vi "Api_GetWaveform.vi"(8 "error in (no error)":errorcluster caption="错误输入（无错误）", 11 "Tags[]":string[](array[string])) -> (0 "error out":errorcluster caption="错误输出", 1 "Display?":bool, 2 "Wave[]":waveform(dbl)[](array[waveform]))   [LabVIEW 2016]
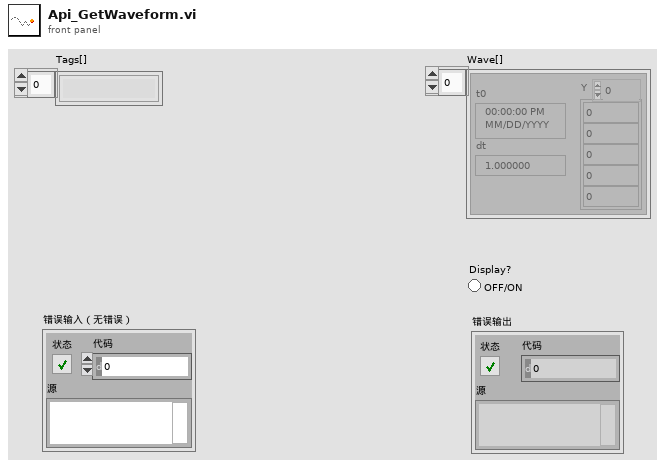
[diagram p1: front panel]
types:
  T1 = cluster{"Queue Name":string, "DAQ Channels":string[], "Queue Type":string}[]
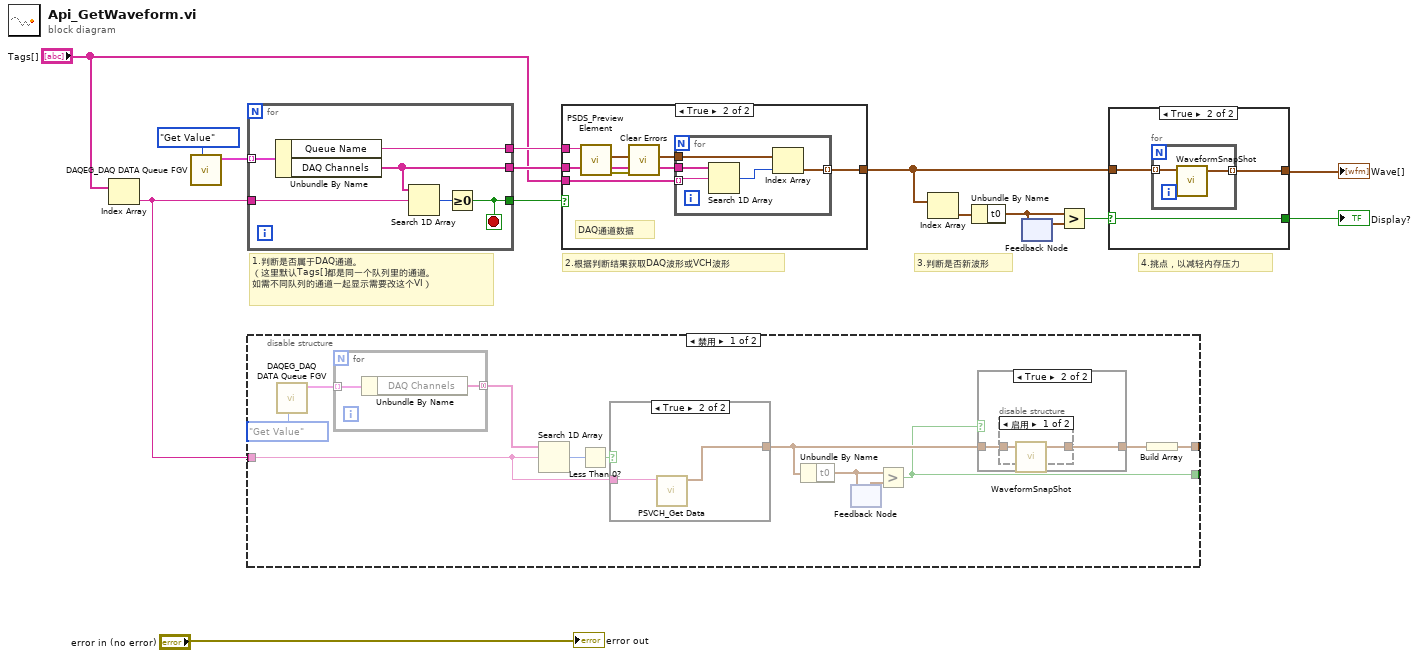
[diagram p0: block diagram]
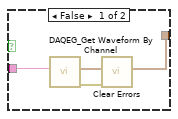
[diagram p2: hidden frame]
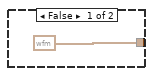
[diagram p3: hidden frame]
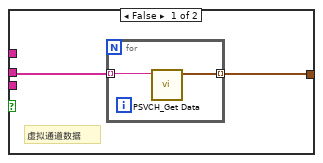
[diagram p7: hidden frame]
diagram:
  # "4.挑点，以减轻内存压力"
  # "3.判断是否新波形"
  # "2.根据判断结果获取DAQ波形或VCH波形"
  # "1.判断是否属于DAQ通道。\n（这里默认Tags[]都是同一个队列里的通道。\n如需不同队列的通道一起显示需要改这个VI）"
  n1 = Index Array(array="Tags[]") -> (element=w12:string)  [unwired: 1 in]
  n2 = call "DAQEG_DAQ DATA Queue FGV.vi"("Command"=enum16{"Initialize", "Get Value", "Set Value"}."Get Value") -> ("DAQ DATA Out"=w13:T1)  [unwired: 9 in, 1 out]
  n3 = for {
    tunnel: w13 -> [w21] mode=indexing
    tunnel: [w20] -> w9
    tunnel: w12 -> [w19]
    tunnel: [w17] -> w11
    tunnel: [w16] -> w10
    stop <- w16 stop-if-true
    n4 = Unbundle By Name(w21) -> ("Queue Name"=w17:string, "DAQ Channels"=w20:string[])
    n5 = Search 1D Array(1D array=w20, element=w19) -> (index of element=w18:i32)  [unwired: 1 in]
    n6 = Greater Or Equal To 0?(x=w18) -> (x >= 0?=w16:bool)
  }
  n7 = disable-structure shown="禁用" {
    disable-tunnel: [w26 _] -> _
    disable-tunnel: [w23 _] -> _
    disable-tunnel: w12 -> [w22 _]
    frame Disabled {
      n8 = call "DAQEG_DAQ DATA Queue FGV.vi"("Command"=enum16{"Initialize", "Get Value", "Set Value"}."Get Value") -> ("DAQ DATA Out"=w27:T1)  [unwired: 9 in, 1 out]
      n9 = for {
        tunnel: w27 -> [w35] mode=indexing
        tunnel: [w34] -> w25 mode=concatenating
        n10 = Unbundle By Name(w35) -> ("DAQ Channels"=w34:string[])
      }
      n11 = Search 1D Array(1D array=w25, element=w22) -> (index of element=w30:i32)  [unwired: 1 in]
      n12 = Less Than 0?(x=w30) -> (x < 0?=w29:bool)
      n13 = case shown="True" w29 {
        tunnel: w22 -> [w38 w40]
        tunnel: [w37 w39] -> w31
        frame False {
          n14 = call "DAQEG_Get Waveform By Channel.vi"("DAQ Channel"=w38) -> ("error out"=w36:errorcluster, "waveform"=w37:waveform(dbl))  [unwired: 9 in]
          n15 = call <vilib>:"Clear Errors.vi"("error in (no error)"=w36) -> ()  [unwired: 5 in, 2 out]
        }
        frame True {
          n16 = call "PSVCH_Get Data.vi"("ChlName"=w40) -> ("Data"=w39:waveform(dbl))  [unwired: 8 in, 2 out]
        }
      }
      n17 = Unbundle By Name(w31) -> ("t0"=w32:timestamp)
      n18 = feedback #1() -> (w33:timestamp)  [unwired: 1 in]
      n19 = feedback-in #1(w32) -> ()
      n20 = Greater?(x=w32, y=w33) -> (0:w26:bool)
      n21 = case shown="True" w26 {
        tunnel: w31 -> [_ w43]
        tunnel: [waveform(dbl) {"t0"=timestamp(0 s since 1904-01-01), "dt"=1.0, "Y"=[]} ("signal out") w42] -> w24
        frame False {
        }
        frame True {
          n22 = disable-structure shown="启用" {
            disable-tunnel: w43 -> [w45 w46]
            disable-tunnel: [w44 w46] -> w42
            frame Enabled {
              n23 = call "WaveformSnapShot.vi"("RawWave"=w45) -> ("SnapWave"=w44:waveform(dbl))  [unwired: 7 in, 1 out]
            }
            frame Disabled {
            }
          }
        }
      }
      n24 = Build Array(w24) -> (w23:waveform(dbl)[])
    }
    frame Enabled {
    }
  }
  n25 = case shown="True" w10 {
    tunnel: w11 -> [_ w56]
    tunnel: w9 -> [w48 w55]
    tunnel: "Tags[]" -> [_ w54]
    tunnel: [w47 w52] -> w4
    frame False {
      # "虚拟通道数据"
      n26 = for {
        tunnel: w48 -> [w50] mode=indexing
        tunnel: [w49] -> w47 mode=indexing
        n27 = call "PSVCH_Get Data.vi"("ChlName"=w50) -> ("Data"=w49:waveform(dbl))  [unwired: 8 in, 2 out]
      }
    }
    frame True {
      # "DAQ通道数据"
      n28 = call "PSDS_Preview Element.vi"("Object Name"=w56) -> ("error out"=w51:errorcluster, "Wave"=w53:waveform(dbl)[])  [unwired: 8 in, 1 out]
      n29 = call <vilib>:"Clear Errors.vi"("error in (no error)"=w51) -> ()  [unwired: 5 in, 2 out]
      n30 = for {
        tunnel: w55 -> [w61]
        tunnel: w54 -> [w60] mode=indexing
        tunnel: w53 -> [w59]
        tunnel: [w57] -> w52 mode=indexing
        n31 = Search 1D Array(1D array=w61, element=w60) -> (index of element=w58:i32)  [unwired: 1 in]
        n32 = Index Array(array=w59, index=w58) -> (element=w57:waveform(dbl))
      }
    }
  }
  n33 = Index Array(array=w4) -> (element=w5:waveform(dbl))  [unwired: 1 in]
  n34 = Unbundle By Name(w5) -> ("t0"=w6:timestamp)
  n35 = feedback #2() -> (w7:timestamp)  [unwired: 1 in]
  n36 = feedback-in #2(w6) -> ()
  n37 = Greater?(x=w6, y=w7) -> (0:w3:bool)
  n38 = case shown="True" w3 {
    selector: w3 -> [w62 w64]
    tunnel: w4 -> [w63 w66]
    tunnel: [w63 w65] -> w2
    tunnel: [w62 w64] -> w1
    frame False {
    }
    frame True {
      n39 = for {
        tunnel: w66 -> [w68] mode=indexing
        tunnel: [w67] -> w65 mode=indexing
        n40 = call "WaveformSnapShot.vi"("RawWave"=w68) -> ("SnapWave"=w67:waveform(dbl))  [unwired: 7 in, 1 out]
      }
    }
  }
  "Display?" <- w1
  "Wave[]" <- w2
  "error out" <- "error in (no error)"
